vi "add transfer group to plugin.vi"(8 "error in (no error)":errorcluster, 9 "transfer group id":string, 10 "id":string, 11 "DSFConfiguration in":refnum<class "DSFConfiguration.lvclass">) -> (0 "error out":errorcluster, 3 "DSFConfiguration out":refnum<class "DSFConfiguration.lvclass">)   [LabVIEW 2017, in "DSFConfiguration.lvclass"]
uses:
  DSFConfiguration.lvclass
  DSFConfiguration.lvclass/DSFConfiguration.ctl
  DSFPlugin/DSFPlugin.lvclass/DSFPlugin.ctl
  DSFPlugin/DSFPlugin.lvclass
  C:/github/data-sharing-framework/Source/Configuration API/Classes/IDable/IDable.lvclass
  DSFGroup/DSFGroup.lvclass
  ID API/ID API.lvclass
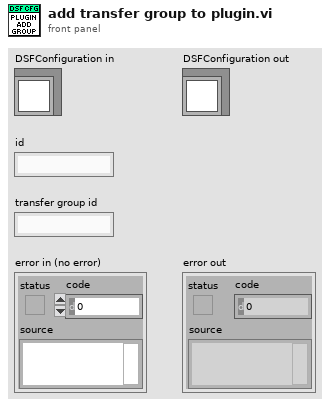
[diagram p1: front panel]
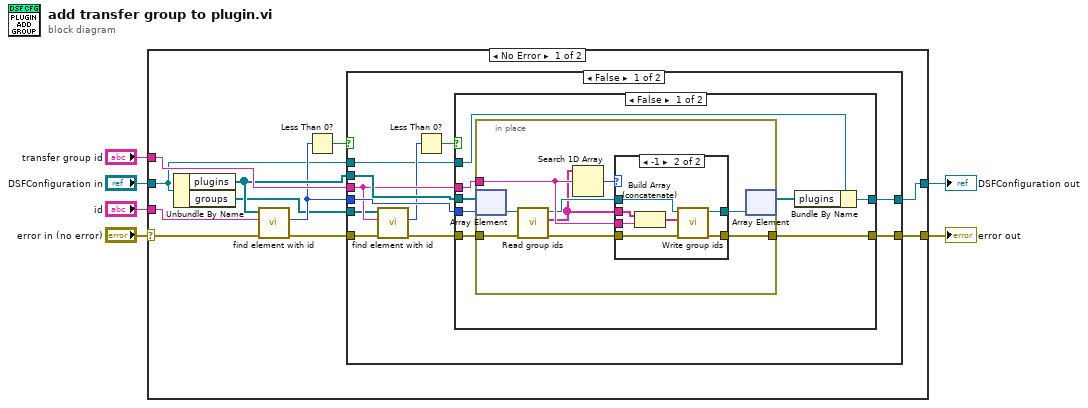
[diagram p0: block diagram]
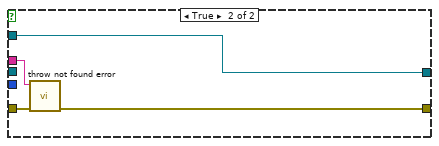
[diagram p3: hidden frame]
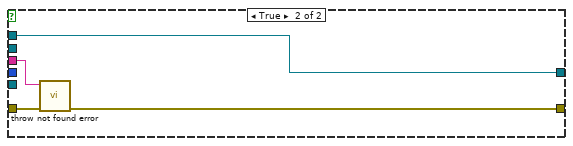
[diagram p4: hidden frame]
diagram:
  n1 = case shown="No Error" "error in (no error)" {
    selector: "error in (no error)" -> [w16 w64]
    tunnel: [w15 w64] -> w5
    tunnel: [w7 w63] -> w3
    tunnel: "DSFConfiguration in" -> [w8 w63]
    tunnel: "id" -> [w17 _]
    tunnel: "transfer group id" -> [w14 _]
    frame No Error {
      n2 = Unbundle By Name(w8) -> ("plugins"=w11:refnum<class "DSFPlugin.lvclass">[], "groups"=w9:refnum<class "DSFGroup.lvclass">[])
      n3 = call "find element with id.vi"("error in (no error)"=w16, "id"=w17, "IDable Array in"=w11) -> ("error out"=w12:errorcluster, "index"=w10:i32)  [unwired: 7 in]
      n4 = Less Than 0?(x=w10) -> (x < 0?=w13:bool)
      n5 = case shown="False" w13 {
        tunnel: w12 -> [w19 w59]
        tunnel: [w26 w62] -> w15
        tunnel: w11 -> [w28 _]
        tunnel: w10 -> [w27 _]
        tunnel: w14 -> [w24 w60]
        tunnel: [w25 w61] -> w7
        tunnel: w9 -> [w23 _]
        tunnel: w8 -> [w20 w61]
        frame False {
          n6 = call "find element with id.vi"("error in (no error)"=w19, "id"=w24, "IDable Array in"=w23) -> ("error out"=w18:errorcluster, "index"=w22:i32)  [unwired: 7 in]
          n7 = Less Than 0?(x=w22) -> (x < 0?=w21:bool)
          n8 = case shown="False" w21 {
            tunnel: w28 -> [w35 _]
            tunnel: w27 -> [w34 _]
            tunnel: w18 -> [w33 w55]
            tunnel: [w31 w58] -> w26
            tunnel: [w30 w57] -> w25
            tunnel: w24 -> [w32 w56]
            tunnel: w20 -> [w29 w57]
            frame False {
              n9 = in-place {
                in-place-border: w32 -> [w43]
                in-place-border: w33 -> [w39]
                in-place-border: [w41] -> w31
                n10 = in-place-array #1(w35, w34) -> (w45:refnum<class "DSFPlugin.lvclass">)
                n11 = call "Read group ids.vi"("error in (no error)"=w39, "DSFPlugin in"=w45) -> ("error out"=w37:errorcluster, "groups ids"=w38:string[], "DSFPlugin out"=w42:refnum<class "DSFPlugin.lvclass">)  [unwired: 7 in]
                n12 = Search 1D Array(1D array=w38, element=w43) -> (index of element=w44:i32)  [unwired: 1 in]
                n13 = case shown="-1" w44 {
                  tunnel: w38 -> [_ w54]
                  tunnel: w43 -> [_ w53]
                  tunnel: w42 -> [w47 w52]
                  tunnel: w37 -> [w46 w48]
                  tunnel: [w46 w51] -> w41
                  tunnel: [w47 w50] -> w40
                  frame Default {
                  }
                  frame -1 {
                    n14 = Build Array (concatenate)(w54, w53) -> (w49:string[])
                    n15 = call "Write group ids.vi"("error in (no error)"=w48, "groups ids"=w49, "DSFPlugin in"=w52) -> ("error out"=w51:errorcluster, "DSFPlugin out"=w50:refnum<class "DSFPlugin.lvclass">)  [unwired: 7 in]
                  }
                }
                n16 = in-place-array #1(w40) -> (w36:refnum<class "DSFPlugin.lvclass">[])  [unwired: 1 out]
              }
              n17 = Bundle By Name(cluster=w29, "plugins"=w36) -> (w30:refnum<class "DSFConfiguration.lvclass">)
            }
            frame True {
              n18 = call "throw not found error.vi"("error in (no error)"=w55, "id"=w56) -> ("error out"=w58:errorcluster)  [unwired: 9 in]
            }
          }
        }
        frame True {
          n19 = call "throw not found error.vi"("error in (no error)"=w59, "id"=w60) -> ("error out"=w62:errorcluster)  [unwired: 9 in]
        }
      }
    }
    frame Error {
    }
  }
  "error out" <- w5
  "DSFConfiguration out" <- w3
